vi "SV Histogram from Buffered Data (DBL) (No State).vi"(0 "data":dbl[](array[numeric]), 5 "range":cluster{"minimum":dbl, "maximum":dbl}={"minimum"=-10.0, "maximum"=10.0}, 7 "number of bins (20)":i32=20) -> (4 "histogram":cluster{"bin centers":dbl[], "counts":u64[]}(graph), 6 "actual range":cluster{"minimum":dbl, "maximum":dbl}={"minimum"=-10.0, "maximum"=10.0}, 8 "counts":T1)   [LabVIEW 2017]
doc: "Use this VI to create a histogram of the input data. Set <B>range</B> and <B>number of bins</B> to specify the bins to include. Choose the appropriate instance based on the input data."
uses:
  <vilib>/addons/_NISVFA/_Shared subVIs/Controls/svc_Histogram Counts.ctl
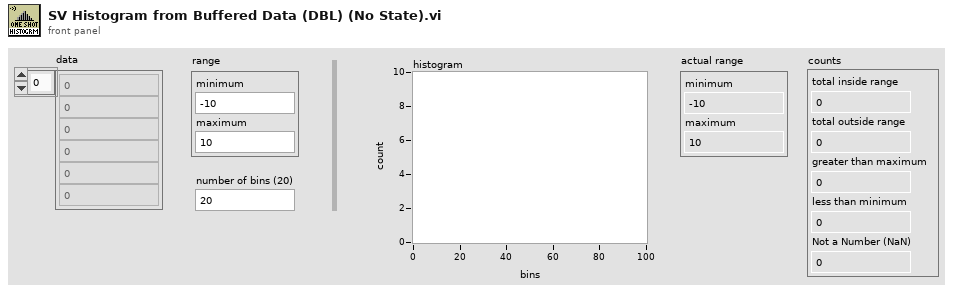
[diagram p1: front panel]
types:
  T1 = typedef "svc_Histogram Counts.ctl" = cluster{"total inside range":u64, "total outside range":u64, "greater than maximum":u64, "less than minimum":u64, "Not a Number (NaN)":u64}
  T2 = typedef "svc_Bin Specification.ctl" = cluster{"lower":dbl, "upper":dbl, "inclusion":u32}
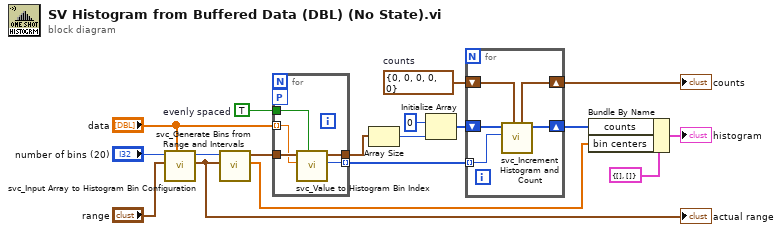
[diagram p0: block diagram]
diagram:
  w2 = TRUE  # evenly spaced
  w9 = T1 {"total inside range"=0, "total outside range"=0, "greater than maximum"=0, "less than minimum"=0, "Not a Number (NaN)"=0}  # counts
  n1 = call <vilib>:"svc_Input Array to Histogram Bin Configuration.vi"("input data"="data", "range in"="range", "number of bins in"="number of bins (20)") -> ("range out"=w11:cluster{"minimum":dbl, "maximum":dbl}, "number of bins out"=w18:i32)  [unwired: 7 in]
  "actual range" <- w11
  n2 = call <vilib>:"svc_Generate Bins from Range and Intervals.vi"("range"=w11, "number of bins"=w18) -> ("nominal centers"=w10:dbl[], "bins"=w7:T2[])  [unwired: 8 in]
  n3 = for {
    tunnel: "data" -> [w21] mode=indexing
    workers-P: _ -> [_]
    tunnel: w7 -> [w23]
    tunnel: [w22] -> w4
    tunnel: w2 -> [w20]
    tunnel: [w19] -> w1 mode=indexing
    n4 = call <vilib>:"svc_Value to Histogram Bin Index.vi"("evenly spaced (F)"=w20, "value"=w21, "bins in"=w23) -> ("bin index"=w19:i32, "bins out"=w22:T2[])  [unwired: 7 in]
  }
  n5 = Array Size(array=w4) -> (size(s)=w15:i32)
  n6 = Initialize Array(u64 0 ("element"), w15) -> (w8:u64[])
  n7 = for {
    shift-right: [w25] -> w5
    shift-left: w8 -> [w26]
    shift-right: [w27] -> w6
    shift-left: w9 -> [w28]
    tunnel: w1 -> [w24] mode=indexing
    n8 = call <vilib>:"svc_Increment Histogram and Count.vi"("counts in"=w28, "bin index"=w24, "histogram in"=w26) -> ("histogram out"=w25:u64[], "counts out"=w27:T1)  [unwired: 7 in]
  }
  "counts" <- w6
  n9 = Bundle By Name(cluster=cluster{"bin centers":dbl[], "counts":u64[]} {"bin centers"=[], "counts"=[]}, "counts"=w5, "bin centers"=w10) -> (→"histogram":cluster{"bin centers":dbl[], "counts":u64[]})
